vi "LED Set.vi"   [LabVIEW 2019]
uses:
  <vilib>/Rock Robotics/WPI/ThirdParty/Phoenix-LabVIEW/CANifier/CTRE_CANifier_LEDChannel.ctl
  LED_States.ctl
  Intake/Intake_Globals.vi
  Globals/Sensor_Values.vi
  Turret/Turret_Globals.vi
  Globals/Magazine_Globals.vi
types:
  T1 = typedef "LED_States.ctl" = enum16{"Off", "Red", "Green", "Yellow", "Blue", "Purple", "Turqoise", "White", "Off Blinking", "Red Blinking", "Green Blinking", "Yellow Blinking", "Blue Blinking", "Purple Blinking", "Turqoise Blinking", "White Blinking"}
  T2 = typedef "CTRE_CANifier_LEDChannel.ctl" = enum32{"LEDChannelA", "LEDChannelB", "LEDChannelC"}
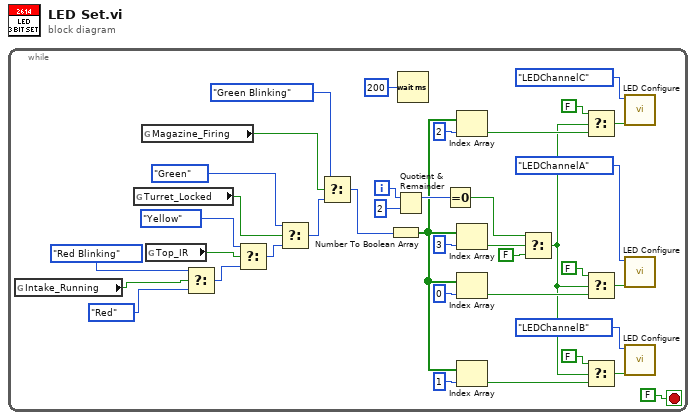
[diagram p0: block diagram]
diagram:
  n1 = while {
    i -> [w32]
    stop <- FALSE stop-if-true
    n2 = global read "Intake_Globals.vi" "Intake_Running"() -> (w12:bool)
    n3 = global read "Turret_Globals.vi" "Turret_Locked"() -> (w5:bool)
    n4 = global read "Magazine_Globals.vi" "Magazine_Firing"() -> (w2:bool)
    n5 = global read "Sensor_Values.vi" "Top_IR"() -> (w9:bool)
    n6 = Select(t=LED_States."Red Blinking" ("LED_States"), s=w12, f=LED_States."Red" ("LED_States")) -> (s? t:f=w10:T1)
    n7 = Select(t=LED_States."Yellow" ("LED_States"), s=w9, f=w10) -> (s? t:f=w7:T1)
    n8 = Select(t=LED_States."Green" ("LED_States"), s=w5, f=w7) -> (s? t:f=w4:T1)
    n9 = Select(t=LED_States."Green Blinking" ("LED_States"), s=w2, f=w4) -> (s? t:f=w3:T1)
    n10 = Number To Boolean Array(number=w3) -> (Boolean array=w19:bool[])
    n11 = Quotient & Remainder(x=w32, y=2) -> (x-y*floor(x/y)=w30:i32)  [unwired: 1 out]
    n12 = Wait (ms)(milliseconds to wait=u32 200) -> ()  [unwired: 1 out]
    n13 = Equal To 0?(x=w30) -> (x = 0?=w17:bool)
    n14 = Index Array(array=w19, index=2) -> (element=w29:bool)
    n15 = Index Array(array=w19, index=3) -> (element=w18:bool)
    n16 = Index Array(array=w19, index=0) -> (element=w22:bool)
    n17 = Index Array(array=w19, index=1) -> (element=w24:bool)
    n18 = Select(t=w17, s=w18, f=FALSE) -> (s? t:f=w16:bool)
    n19 = Select(t=FALSE, s=w16, f=w29) -> (s? t:f=w26:bool)
    n20 = Select(t=FALSE, s=w16, f=w22) -> (s? t:f=w21:bool)
    n21 = Select(t=FALSE, s=w16, f=w24) -> (s? t:f=w25:bool)
    n22 = call "LED Configure.vi"("LED On"=w26, "LEDChannel"=CTRE_CANifier_LEDChannel."LEDChannelC") -> ()  [unwired: 10 in]
    n23 = call "LED Configure.vi"("LED On"=w21, "LEDChannel"=CTRE_CANifier_LEDChannel."LEDChannelA") -> ()  [unwired: 10 in]
    n24 = call "LED Configure.vi"("LED On"=w25, "LEDChannel"=CTRE_CANifier_LEDChannel."LEDChannelB") -> ()  [unwired: 10 in]
  }
